vi "testParseNotReadingModifiedDataProperly(Case5788).vi"(8 "error in (no error)":errorcluster, 11 "reference in":refnum<class "EasyXMLTest.lvclass">) -> (0 "error out":errorcluster, 3 "reference in":refnum<class "EasyXMLTest.lvclass">)   [LabVIEW 2013, in "EasyXMLTest.lvclass"]
uses:
  EasyXMLTest.lvclass
panel:
  in  "sequence":T1={"version"=1.0, "test"="hello", "new feature"=0.0}
  out "sequence":T1
  in  "XML String":string="<sequence>\r\n  <version>1</version>\r\n  <test>hello</test>\r\n</sequence>"
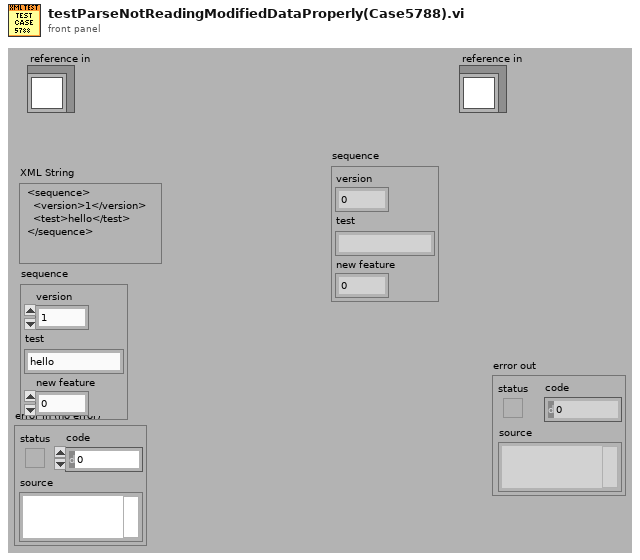
[diagram p1: front panel]
types:
  T1 = cluster{"version":dbl, "test":string, "new feature":dbl}
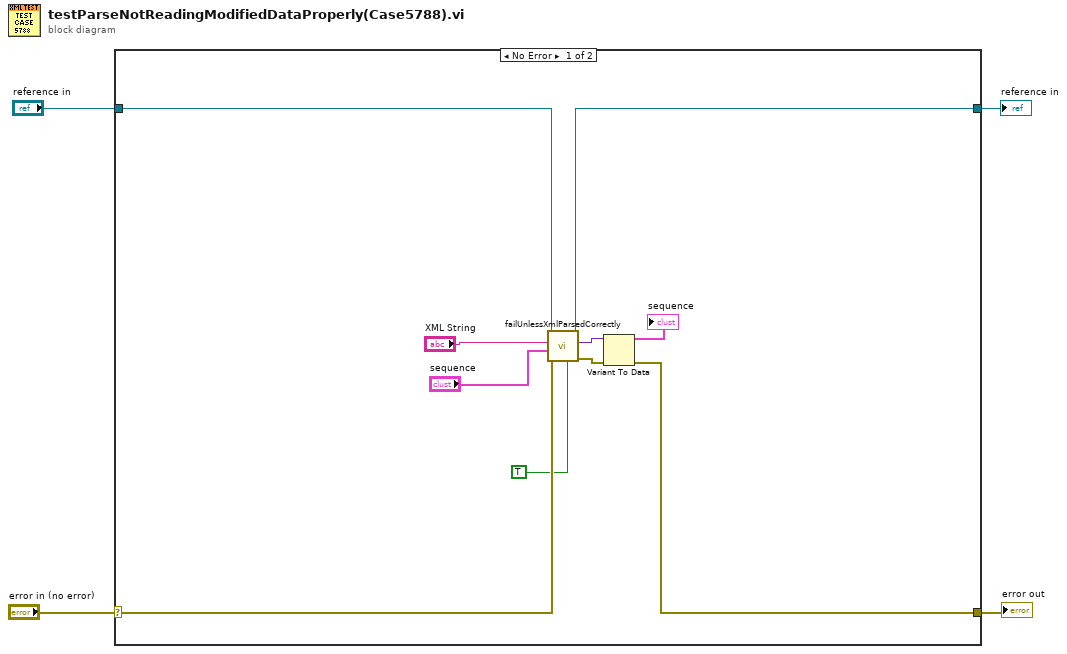
[diagram p0: block diagram]
diagram:
  n1 = case shown="No Error" "error in (no error)" {
    selector: "error in (no error)" -> [w12 w16]
    tunnel: [w5 w16] -> w3
    tunnel: [w13 w15] -> w1
    tunnel: "reference in" -> [w14 w15]
    frame No Error {
      n2 = call "failUnlessXmlParsedCorrectly.vi"("Convert EOL? (TRUE)"=TRUE, "error in"=w12, "Expected Data"="sequence", "XML String"="XML String", "reference in"=w14) -> ("error out"=w6:errorcluster, "Produced Data"=w10:variant, "reference in"=w13:refnum<class "EasyXMLTest.lvclass">)  [unwired: 4 in]
      n3 = Variant To Data(error in=w6, Variant=w10) -> (data=→"sequence":T1, error out=w5:errorcluster)  [unwired: 1 in]
    }
    frame Error {
    }
  }
  "error out" <- w3
  "reference in" <- w1
